vi "init.vi"(8 "error in":errorcluster, 10 "TBM module configuration in":refnum<class "TBM module configuration.lvclass">, 11 "Shared Library Module runtime in":refnum<class "Shared Library Module runtime.lvclass">) -> (0 "error out":errorcluster, 1 "data allocations":T1, 2 "execution settings":T4, 3 "Shared Library Module runtime out":refnum<class "Shared Library Module runtime.lvclass">)   [LabVIEW 2013, in "Shared Library Module runtime.lvclass"]
doc: "Provides an interface for initializing a module at runtime. While this interface performs no operations, a child should provide an override which may open any necessary references or sessions, allocate necessary memory, and perform any final configuration validataion before providing the full configuration <b>execution data</b> to the calling process.Platypus Framework 1.0.1.60\nNI Systems Engineering - National Instruments"
uses:
  Shared Library Module runtime.lvclass
  <vilib>/NI/Tag Bus Module Framework/module configuration/TBM module configuration.lvclass
  <vilib>/NI/Tag Bus Module Framework/runtime/execution settings.ctl
  <vilib>/NI/Tag Bus Module Framework/channel/data tables.ctl
  <vilib>/NI/Tag Bus/dictionary/data dictionary.lvclass
  <vilib>/NI/Tag Bus/dictionary table pair.ctl
  <vilib>/NI/Tag Bus/table/data table.ctl
  configuration/Shared Library Module configuration.lvclass
  configuration/Shared Library Module configuration.lvclass/Shared Library Module configuration.ctl
  Shared Library Module runtime.lvclass/Shared Library Module runtime.ctl
  configuration/Read dllpath.vi
  configuration/Read args.vi
  <vilib>/NI/Tag Bus Module Framework/runtime/TBM module execution interface.lvclass
  <vilib>/NI/Tag Bus Module Framework/channel/TBM channel.lvclass
  <vilib>/NI/Tag Bus/tag bus.lvlib
  <vilib>/NI/Tag Bus/table/data table.lvlib
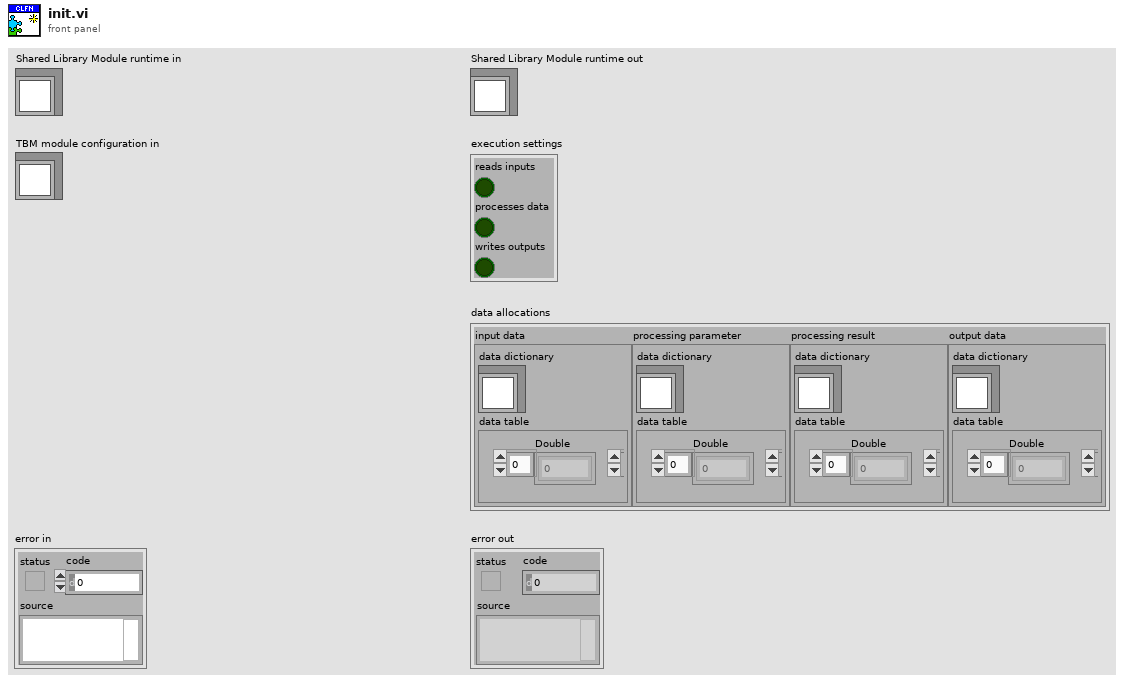
[diagram p1: front panel]
types:
  T1 = typedef "TBM channel.lvclass/data tables.ctl" = cluster{"input data":T2, "processing parameter":T2, "processing result":T2, "output data":T2}
  T2 = typedef "tag bus.lvlib/dictionary table pair.ctl" = cluster{"data dictionary":refnum<class "data dictionary.lvclass">, "data table":T3}
  T3 = typedef "tag bus.lvlib/data table.lvlib/data table.ctl" = cluster{"Double":dbl[], "Single":sgl[], "I64":i64[], "I32":i32[], "I16":i16[], "I8":i8[], "U64":u64[], "U32":u32[], "U16":u16[], "U8":u8[], "Boolean":bool[], "String":string[], "Array of Double":cluster{"DBL Array":dbl[]}[], "Array of Single":cluster{"SGL Array":sgl[]}[], "Array of I64":cluster{"I64 Array":i64[]}[], "Array of I32":cluster{"I32 Array":i32[]}[], "Array of I16":cluster{"I16 Array":i16[]}[], "Array of I8":cluster{"I8 Array":i8[]}[], "Array of U64":cluster{"U64 Array":u64[]}[], "Array of U32":cluster{"U32 Array":u32[]}[], "Array of U16":cluster{"U16 Array":u16[]}[], "Array of U8":cluster{"U8 Array":u8[]}[], "Array of Boolean":cluster{"Boolean Array":bool[]}[], "Array of String":cluster{"String Array":string[]}[]}
  T4 = typedef "TBM module execution interface.lvclass/execution settings.ctl" = cluster{"reads inputs":bool, "processes data":bool, "writes outputs":bool}
  T5 = typedef "tag bus.lvlib/data dictionary.lvclass/full data dictionary.ctl" = cluster{"Double":string[], "Single":string[], "I64":string[], "I32":string[], "I16":string[], "I8":string[], "U64":string[], "U32":string[], "U16":string[], "U8":string[], "Boolean":string[], "String":string[], "Array of Double":string[], "Array of Single":string[], "Array of I64":string[], "Array of I32":string[], "Array of I16":string[], "Array of I8":string[], "Array of U64":string[], "Array of U32":string[], "Array of U16":string[], "Array of U8":string[], "Array of Boolean":string[], "Array of String":string[]}
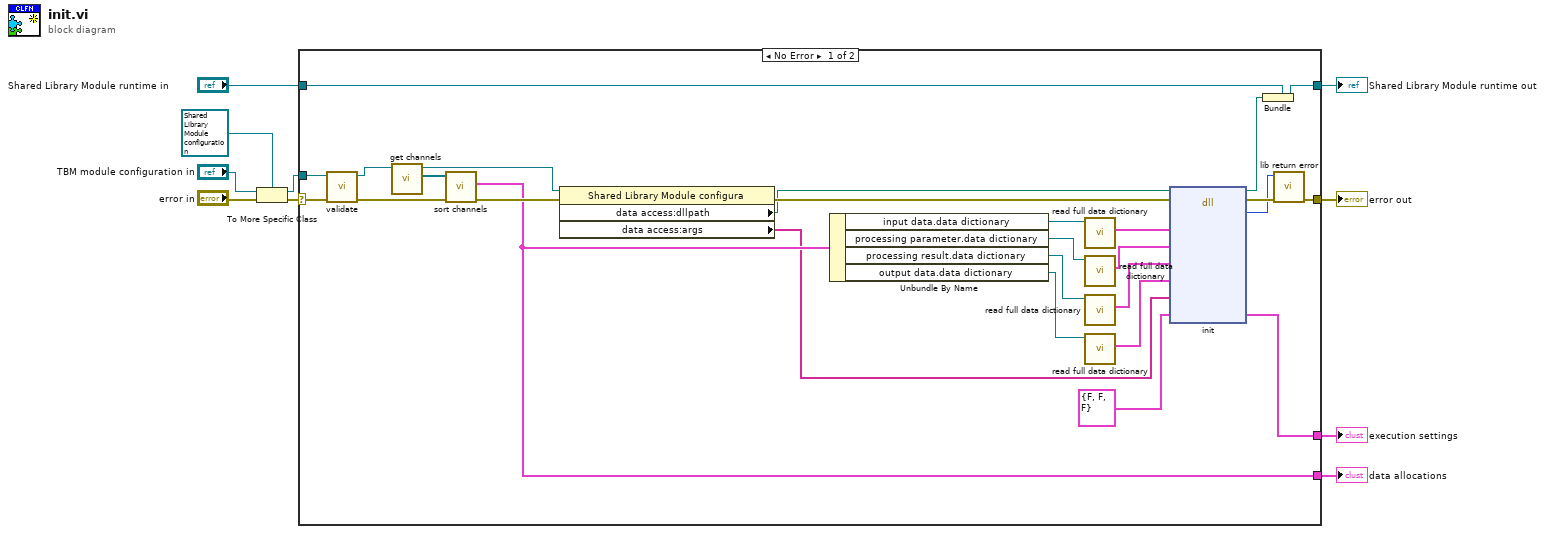
[diagram p0: block diagram]
diagram:
  n1 = To More Specific Class(target class=refnum<class "Shared Library Module configuration.lvclass"> refnum ("Synchronous module configuration"), reference="TBM module configuration in", error in="error in") -> (specific class reference=w6:refnum<class "Shared Library Module configuration.lvclass">, error out=w7:errorcluster)
  n2 = case shown="No Error" w7 {
    selector: w7 -> [w34 w38]
    tunnel: w6 -> [w33 _]
    tunnel: "Shared Library Module runtime in" -> [w37 w39]
    tunnel: [w30 w39] -> w4
    tunnel: [w11 w38] -> w3
    tunnel: [w16 _] -> w1
    tunnel: [w17 _] -> w2
    frame No Error {
      n3 = call-dynamic "validate.vi"("error in"=w34, "Shared Library Module configuration in"=w33) -> ("error out"=w35:errorcluster, "Shared Library Module configuration out"=w32:refnum<class "Shared Library Module configuration.lvclass">)  [unwired: 8 in]
      n4 = call-dynamic "get channels.vi"("Shared Library Module configuration in"=w32) -> ("channels"=w31:refnum<class "TBM channel.lvclass">[], "Shared Library Module configuration out"=w29:refnum<class "Shared Library Module configuration.lvclass">)  [unwired: 9 in]
      n5 = call <vilib>:"sort channels.vi"("error in"=w35, "channels in"=w31) -> ("error out"=w36:errorcluster, "data allocations"=w16:T1)  [unwired: 7 in, 1 out]
      n6 = property class="Shared Library Module configura"(reference=w29, error in=w36) -> (error out=w19:errorcluster, "data access:dllpath"=w15:path, "data access:args"=w14:string[])  [unwired: 1 out]
      n7 = Unbundle By Name(w16) -> ("input data.data dictionary"=w24:refnum<class "data dictionary.lvclass">, "processing parameter.data dictionary"=w25:refnum<class "data dictionary.lvclass">, "processing result.data dictionary"=w26:refnum<class "data dictionary.lvclass">, "output data.data dictionary"=w27:refnum<class "data dictionary.lvclass">)
      n8 = call <vilib>:"read full data dictionary.vi"("data dictionary in"=w24) -> ("dictionary"=w23:T5)  [unwired: 8 in, 2 out]
      n9 = call <vilib>:"read full data dictionary.vi"("data dictionary in"=w25) -> ("dictionary"=w22:T5)  [unwired: 8 in, 2 out]
      n10 = call <vilib>:"read full data dictionary.vi"("data dictionary in"=w26) -> ("dictionary"=w21:T5)  [unwired: 8 in, 2 out]
      n11 = call <vilib>:"read full data dictionary.vi"("data dictionary in"=w27) -> ("dictionary"=w20:T5)  [unwired: 8 in, 2 out]
      n12 = dll-call lib="?" fn="init"(path in=w15, error in=w19, "idict"=w23, "pdict"=w22, "rdict"=w21, "odict"=w20, "args"=w14, "execSettings"=T4 {"reads inputs"=FALSE, "processes data"=FALSE, "writes outputs"=FALSE} ("execution settings")) -> (path out=w18:path, error out=w13:errorcluster, "return type"=w12:i32, "execSettings"=w17:T4)  [unwired: 6 in]
      n13 = Bundle(cluster=w37, w18) -> (w30:refnum<class "Shared Library Module runtime.lvclass">)
      n14 = call "lib return error.vi"("error in"=w13, "return value"=w12) -> ("error out"=w11:errorcluster)  [unwired: 9 in]
    }
    frame Error {
    }
  }
  "error out" <- w3
  "Shared Library Module runtime out" <- w4
  "execution settings" <- w2
  "data allocations" <- w1
